vi "Savitsky Golay Weighted Filter (multiple).vi"(4 "Window Order":i32, 6 "Side Points Unit (points)":enum16{"Points", "Data"}(ring), 8 "error in (no error)":errorcluster, 9 "polynomial order (3)":i32=3, 10 "side points (6)":dbl=6.0, 11 "XY-data":cluster{"X-array":dbl[], "Y-array":dbl[]}[](array[cluster])) -> (0 "error out":errorcluster, 3 "XY-data out":cluster{"X-array":dbl[], "Y-array":dbl[]}[](array[cluster]) {"Y-array" format="%.2p"; "X-array" format="%.2p"})   [LabVIEW 2019, in "xy_utilities.lvlib"]
doc: "Filter <b>XY-data</b>'s Y-Array with a Savitsky-Golay FIR smoothing filter.\n\n<b>side points</b> specifies the number of data points to each side of the current data point to use for the least squares minimization. side points*2 + 1 is the length of the moving window, which must be greater than the polynomial order.\n\n<b>polynomial order</b> specifies the order of the polynomial. \n\nWire data to the data input to determine the polymorphic instance to use or manually select the instance."
uses:
  xy_utilities.lvlib
  Private/X Units.vi
  <vilib>/Analysis/3filter.llb/Savitzky-Golay Filter.vi
  <vilib>/Analysis/3filter.llb/Savitzky-Golay Filter (DBL).vi
  Private/X Array Range to Index.vi
  Private/Hann Windows.vi
  <vilib>/Utility/error.llb/Error Cluster From Error Code.vi
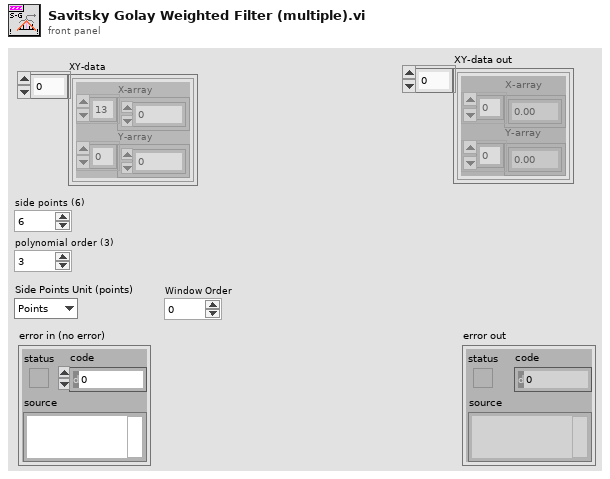
[diagram p1: front panel]
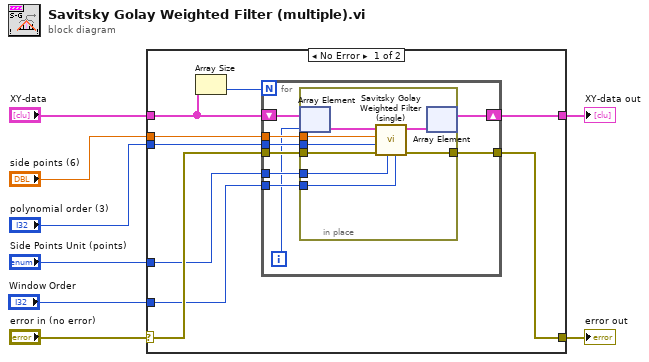
[diagram p0: block diagram]
diagram:
  n1 = case shown="No Error" "error in (no error)" {
    selector: "error in (no error)" -> [w15 w36]
    tunnel: [w14 w36] -> w7
    tunnel: "XY-data" -> [w9 w35]
    tunnel: [w17 w35] -> w5
    tunnel: "side points (6)" -> [w16 _]
    tunnel: "polynomial order (3)" -> [w13 _]
    tunnel: "Window Order" -> [w12 _]
    tunnel: "Side Points Unit (points)" -> [w11 _]
    frame No Error {
      n2 = Array Size(array=w9) -> (size(s)=w10:i32)
      n3 = for {
        N: w10 -> [_]
        tunnel: w16 -> [w26]
        tunnel: w15 -> [w25]
        tunnel: [w24] -> w14
        tunnel: w11 -> [w21]
        tunnel: w13 -> [w23]
        tunnel: w12 -> [w22]
        shift-right: [w18] -> w17
        shift-left: w9 -> [w20]
        i -> [w19]
        n4 = in-place {
          in-place-border: w26 -> [w34]
          in-place-border: w25 -> [w33]
          in-place-border: [w32] -> w24
          in-place-border: w23 -> [w31]
          in-place-border: w22 -> [w30]
          in-place-border: w21 -> [w29]
          n5 = in-place-array #1(w20, w19) -> (w28:cluster{"X-array":dbl[], "Y-array":dbl[]})
          n6 = call "Savitsky Golay Weighted Filter (single).vi"("Window Order"=w30, "Side Points Unit (points)"=w29, "error in (no error)"=w33, "polynomial order (3)"=w31, "side points (6)"=w34, "XY-data"=w28) -> ("error out"=w32:errorcluster, "XY-data out"=w27:cluster{"X-array":dbl[], "Y-array":dbl[]})  [unwired: 4 in]
          n7 = in-place-array #1(w27) -> (w18:cluster{"X-array":dbl[], "Y-array":dbl[]}[])  [unwired: 1 out]
        }
      }
    }
    frame Error {
    }
  }
  "error out" <- w7
  "XY-data out" <- w5
